vi "GetDecorationLocation.vi"(6 "error in":errorcluster, 9 "Decoration in":refnum<class "Decoration.lvclass">) -> (0 "error out":errorcluster, 3 "Decoration out":refnum<class "Decoration.lvclass">, 4 "Position":T1)   [LabVIEW 2014, in "Decoration.lvclass"]
uses:
  Decoration.lvclass
  <vilib>/Utility/miscctls.llb/LVPositionTypeDef.ctl
  GObject/GObject.lvclass/GObject.ctl
  GObject/GObject.lvclass
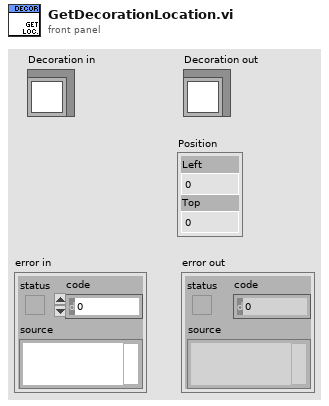
[diagram p1: front panel]
types:
  T1 = typedef "LVPositionTypeDef.ctl" = cluster{"Left":i32, "Top":i32}
  T2 = typedef "LVRectTypeDef.ctl" = cluster{"Left":i16, "Top":i16, "Right":i16, "Bottom":i16}
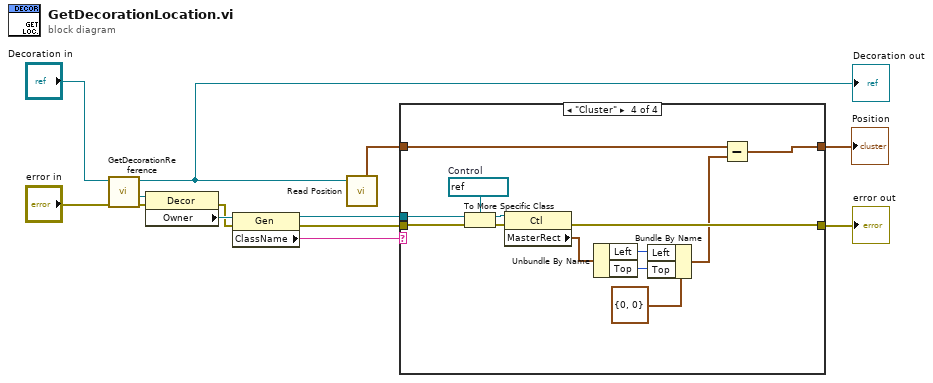
[diagram p0: block diagram]
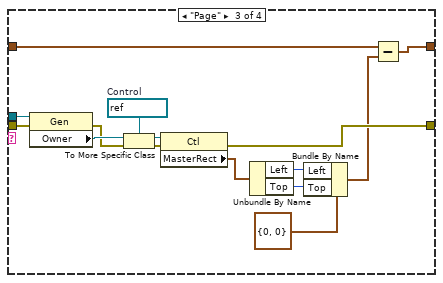
[diagram p4: hidden frame]
diagram:
  n1 = call "GetDecorationReference.vi"("error in"="error in", "Decoration in"="Decoration in") -> ("error out"=w10:errorcluster, "Decoration reference"=w11:refnum<vi>, "Decoration out"=w2:refnum<class "Decoration.lvclass">)  [unwired: 7 in]
  "Decoration out" <- w2
  n2 = property class="Decor"(reference=w11, error in=w10) -> (error out=w8:errorcluster, "Owner"=w9:refnum<vi>)  [unwired: 1 out]
  n3 = property class="Gen"(reference=w9, error in=w8) -> (reference out=w6:refnum<vi>, error out=w1:errorcluster, "ClassName"=w7:string)
  n4 = call "Read Position.vi"("GObject in"=w2) -> ("Position"=w5:T1)  [unwired: 7 in, 1 out]
  n5 = case shown="\"Cluster\"" w7 {
    tunnel: [w14 w16 w23 w35] -> w3
    tunnel: w6 -> [_ _ w32 w42]
    tunnel: w5 -> [w15 w17 w28 w44]
    tunnel: [w15 w17 w27 w43] -> w4
    tunnel: w1 -> [w14 w16 w26 w41]
    frame Default {
    }
    frame "Panel" {
    }
    frame "Page" {
      w31 = refnum<vi> refnum  # Control
      n6 = property class="Gen"(reference=w32, error in=w26) -> (error out=w29:errorcluster, "Owner"=w30:refnum<vi>)  [unwired: 1 out]
      n7 = To More Specific Class(target class=w31, reference=w30, error in=w29) -> (specific class reference=w25:refnum<vi>, error out=w24:errorcluster)
      n8 = property class="Ctl"(reference=w25, error in=w24) -> (error out=w23:errorcluster, "MasterRect"=w22:T2)  [unwired: 1 out]
      n9 = Unbundle By Name(w22) -> ("Left"=w21:i16, "Top"=w20:i16)
      n10 = Bundle By Name(cluster=T1 {"Left"=0, "Top"=0} ("Position"), "Left"=w21, "Top"=w20) -> (w19:T1)
      n11 = Subtract(x=w28, y=w19) -> (x-y=w27:T1)
    }
    frame "Cluster" {
      w45 = refnum<vi> refnum  # Control
      n12 = To More Specific Class(target class=w45, reference=w42, error in=w41) -> (specific class reference=w37:refnum<vi>, error out=w36:errorcluster)
      n13 = property class="Ctl"(reference=w37, error in=w36) -> (error out=w35:errorcluster, "MasterRect"=w40:T2)  [unwired: 1 out]
      n14 = Unbundle By Name(w40) -> ("Left"=w39:i16, "Top"=w38:i16)
      n15 = Bundle By Name(cluster=T1 {"Left"=0, "Top"=0} ("Position"), "Left"=w39, "Top"=w38) -> (w33:T1)
      n16 = Subtract(x=w44, y=w33) -> (x-y=w43:T1)
    }
  }
  "error out" <- w3
  "Position" <- w4
